vi "PWM-PID-ENCODER LIFA  - PID original  -Kalman filter test + PID  test new period of pid - Copie.vi"() -> ()   [LabVIEW 2018]
uses:
  <vilib>/LabVIEW Interface for Arduino/Type Defs/Board Type.ctl
  Control 1.ctl
  <vilib>/LabVIEW Interface for Arduino/Type Defs/Pin Mode.ctl
  <vilib>/Analysis/Matrix/Datatypes/RealMatrix.ctl
  <vilib>/addons/control/pid/pid.llb/PID (DBL).vi
  <vilib>/LabVIEW Interface for Arduino/LabVIEW Interface for Arduino.lvlib
  <vilib>/Analysis/Matrix/NI_Matrix.lvlib
  <vilib>/addons/control/pid/NI_PID_pid.lvlib
panel:
  in  "?":enum32{"Page 1", "Page 2"}(tab)
  in  "STOP":bool
  in  "RESET":bool
  in  "USB  COM":refnum<visa-resource-name>="COM12"
  in  "Platforme":T1
  in  "Direction 1":bool
  in  "Direction 2":bool
  in  "gains PID":T2={"Proportional gain (Kc)"=1.0, "Integral  (Ti )"=0.01, "Derivative  (Td)"=0.0} {"Derivative  (Td)" scale=0.0..30.0; "Integral  (Ti )" scale=0.0..30.0; "Proportional gain (Kc)" scale=0.0..30.0}
  in  "Consigne":dbl(knob) scale=0.0..1500.0
  out "PWM(%)":dbl(slide) scale=0.0..100.0
  out "Vitesse":T3
  in  "Contrôle manuel":dbl(knob) scale=100.0..255.0
  in  "Mode":bool
  out "Estimation de vitesse":cluster{"Real Matrix Element":dbl, dbl}(graph) caption="Waveform Chart"
  out "Vitesse  (tr/min)":dbl(knob) scale=0.0..1500.0
  # "Tableau de Bord"
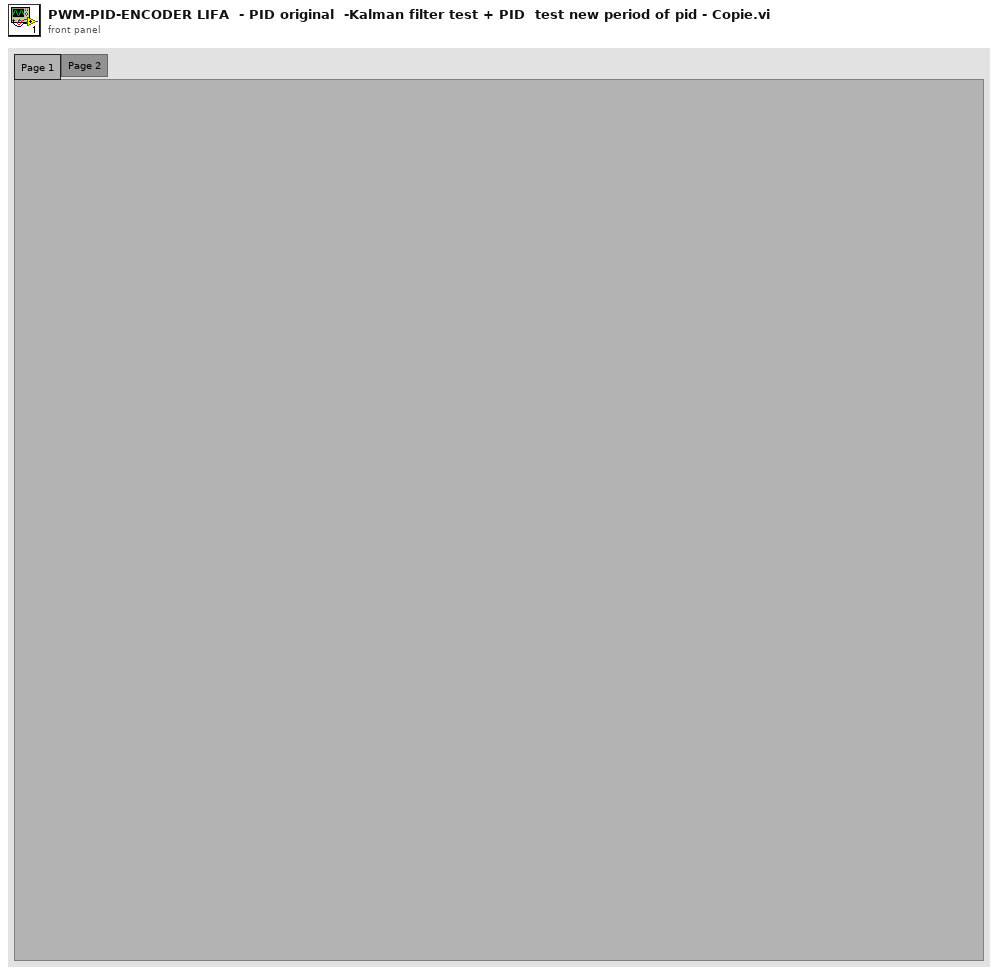
[diagram p1: front panel]
types:
  T1 = typedef "LabVIEW Interface for Arduino.lvlib/Board Type.ctl" = enum16{"Uno", "Dimuelanove w/Atmega 328", "Mega 2560"}
  T2 = cluster{"Proportional gain (Kc)":dbl, "Integral  (Ti )":dbl, "Derivative  (Td)":dbl}
  T3 = typedef "Control 1.ctl" = dynamicdata
  T4 = typedef "LabVIEW Interface for Arduino.lvlib/Pin Mode.ctl" = enum8{"Input", "Output"}
  T5 = typedef "LabVIEW Interface for Arduino.lvlib/Arduino Resource.ctl" = cluster{"VISA resource":refnum<visa-resource-name>, "Board Type":T1, "Connection Type":enum8{"USB / Serial"}, "Bytes Per Packet (15)":u8}
  T6 = typedef "NI_Matrix.lvlib/RealMatrix.ctl" = dbl[][]
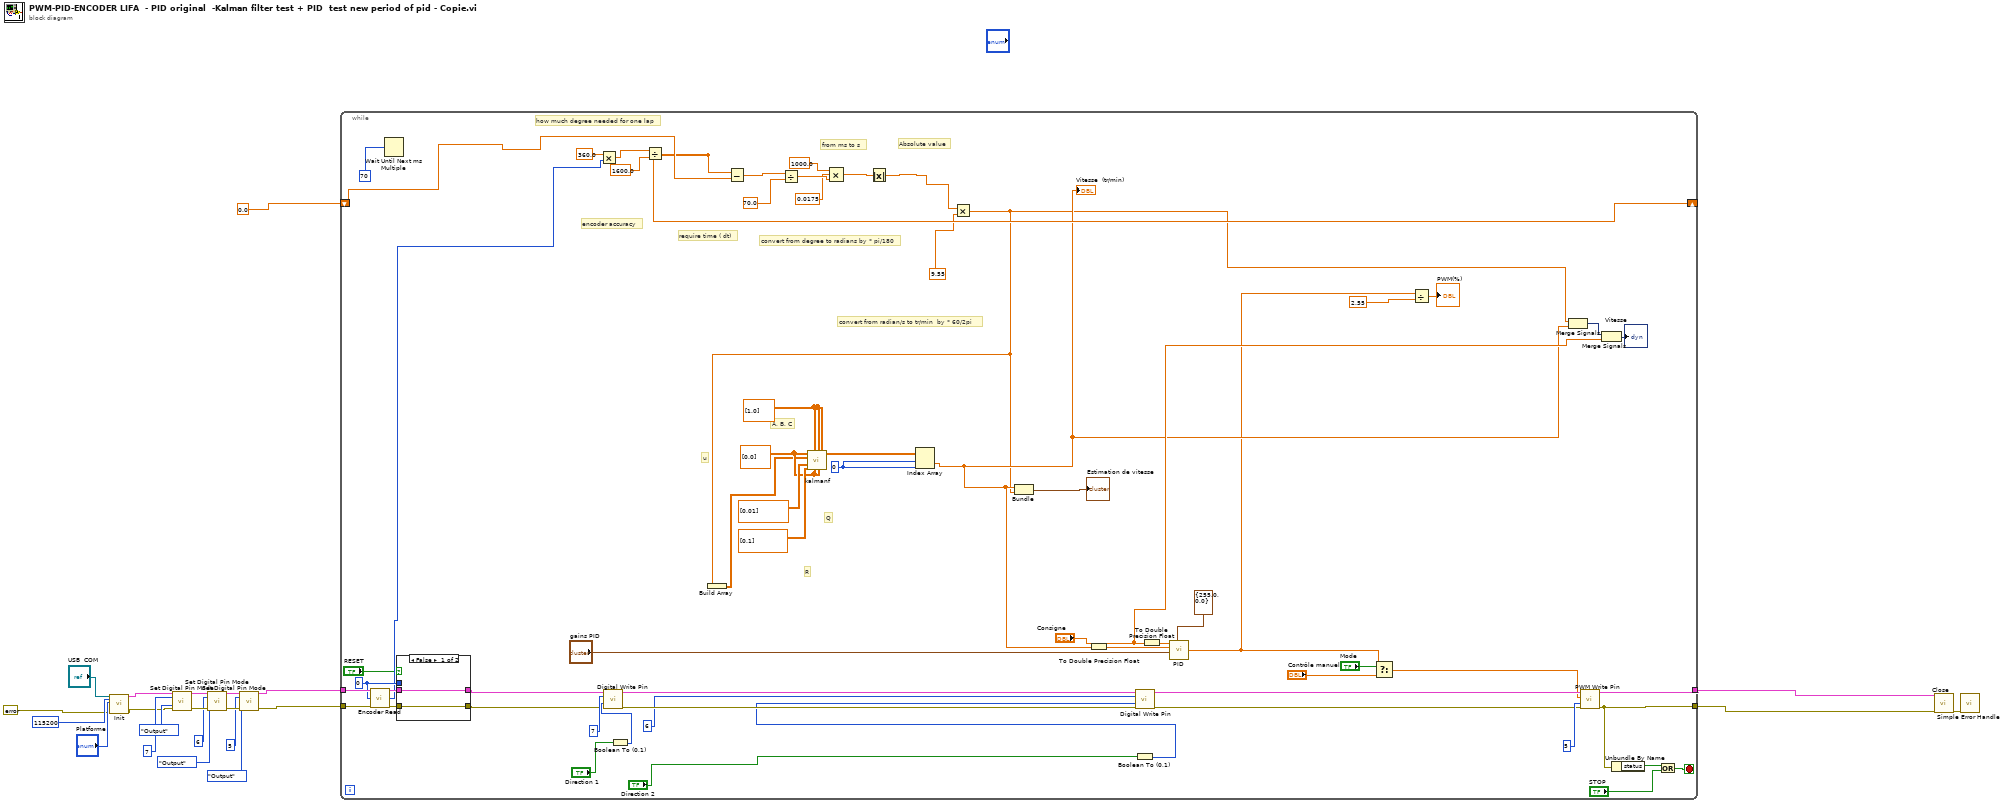
[diagram p0: block diagram]
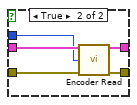
[diagram p2: hidden frame]
diagram:
  n1 = call <vilib>:"Init.vi"("VISA resource"="USB  COM", "Baud Rate (115200)"=u32 115200, "Board Type (Uno)"="Platforme", "error in"=errorcluster {"status"=FALSE, "code"=0, "source"=""}) -> ("Arduino Resource"=w7:T5, "error out"=w6:errorcluster)  [unwired: 14 in]
  n2 = call <vilib>:"Set Digital Pin Mode.vi"("Arduino Resource"=w7, "Digital I/O Pin"=u8 7, "Pin Mode (Input)"=Pin_Mode."Output", "error in"=w6) -> ("Arduino Resource"=w17:T5, "error out"=w16:errorcluster)  [unwired: 10 in]
  n3 = call <vilib>:"Set Digital Pin Mode.vi"("Arduino Resource"=w17, "Digital I/O Pin"=u8 6, "Pin Mode (Input)"=Pin_Mode."Output", "error in"=w16) -> ("Arduino Resource"=w15:T5, "error out"=w14:errorcluster)  [unwired: 10 in]
  n4 = call <vilib>:"Set Digital Pin Mode.vi"("Arduino Resource"=w15, "Digital I/O Pin"=u8 5, "Pin Mode (Input)"=Pin_Mode."Output", "error in"=w14) -> ("Arduino Resource"=w5:T5, "error out"=w4:errorcluster)  [unwired: 10 in]
  n5 = while {
    tunnel: w5 -> [w84]
    tunnel: w4 -> [w81]
    tunnel: [w64] -> w22
    tunnel: [w65] -> w2
    shift-right: [w29] -> _
    shift-left: 0.0 -> [w31]
    stop <- w80 stop-if-true
    w46 = 0 ("index (row)")
    w48 = T6 [[0.0]] ("U")
    w51 = T6 [[1.0]] ("A")
    w78 = u8 0 ("Encoder Number (0)")
    # "Absolute value"
    # "convert from radian/s to tr/min  by * 60/2pi"
    # "how much degree needed for one lap"
    # "encoder accuracy"
    # "from ms to s"
    # "require time ( dt)"
    # "convert from degree to radians by * pi/180"
    # "A, B, C"
    # "R"
    # "Q"
    # "u"
    n6 = call "Encoder Read.vi"("Arduino Resource"=w84, "Encoder Number (0)"=w78, "error in"=w81) -> ("Arduino Resource Out"=w83:T5, "Count"=w32:i32, "error out"=w82:errorcluster)  [unwired: 10 in]
    n7 = Wait Until Next ms Multiple(millisecond multiple=u32 70) -> ()  [unwired: 1 out]
    n8 = case shown="False" "RESET" {
      tunnel: w83 -> [w86 w91]
      tunnel: [w86 w90] -> w63
      tunnel: [w85 w89] -> w62
      tunnel: w82 -> [w85 w88]
      tunnel: w78 -> [_ w87]
      frame False {
      }
      frame True {
        n9 = call "Encoder Read.vi"("Arduino Resource"=w91, "Encoder Number (0)"=w87, "error in"=w88) -> ("Arduino Resource Out"=w90:T5, "error out"=w89:errorcluster)  [unwired: 10 in, 1 out]
      }
    }
    n10 = Multiply(x=360.0, y=w32) -> (x*y=w39:dbl)
    n11 = Boolean To (0,1)(Boolean="Direction 1") -> (0, 1=w69:i16)
    n12 = call <vilib>:"Digital Write Pin.vi"("Arduino Resource"=w63, "Digital I/O Pin (0)"=u8 7, "Value (0)"=w69, "error in"=w62) -> ("Arduino Resource"=w75:T5, "error out"=w74:errorcluster)  [unwired: 10 in]
    n13 = Divide(x=w39, y=1600.0) -> (x/y=w29:dbl)
    n14 = Subtract(x=w29, y=w31) -> (x-y=w37:dbl)
    n15 = Divide(x=w37, y=70.0) -> (x/y=w35:dbl)
    n16 = Compound Arithmetic op=MULTIPLY(1000.0 ("value"), 0.0175 ("value"), w35) -> (w28:dbl)
    n17 = Absolute Value(x=w28) -> (abs(x)=w26:dbl)
    n18 = Multiply(x=w26, y=9.55) -> (x*y=w24:dbl)
    n19 = Build Array(w24) -> (w47:T6)
    n20 = call "kalmanf.vi"("u"=w48, "A"=w51, "B"=w51, "C"=w51, "y"=w47, "Q"=T6 [[0.01]], "R"=T6 [[0.1]] ("Q"), "xhat0"=w48, "P0"=w48) -> ("xhat"=w45:T6)  [unwired: 6 in]
    n21 = Index Array(array=w45, index (row)=w46, index (col)=w46) -> (element=w25:dbl)
    "Vitesse  (tr/min)" <- w25
    n22 = Bundle("Real Matrix Element"=w25, w24) -> (→"Estimation de vitesse":cluster{"Real Matrix Element":dbl, dbl})  [unwired: 1 in]
    n23 = To Double Precision Float(number=w25) -> (double precision float=w59:dbl)
    n24 = Boolean To (0,1)(Boolean="Direction 2") -> (0, 1=w67:i16)
    n25 = call <vilib>:"Digital Write Pin.vi"("Arduino Resource"=w75, "Digital I/O Pin (0)"=u8 6, "Value (0)"=w67, "error in"=w74) -> ("Arduino Resource"=w73:T5, "error out"=w72:errorcluster)  [unwired: 10 in]
    n26 = To Double Precision Float(number="Consigne") -> (double precision float=w42:dbl)
    n27 = call-poly <vilib>:"PID.vi"("output range"=cluster{"output high":dbl, "output low":dbl} {"output high"=255.0, "output low"=0.0}, "PID gains"="gains PID", "process variable"=w59, "setpoint"=w42) -> ("output"=w23:dbl)  [unwired: 6 in, 1 out]
    n28 = Select(t=w23, s="Mode", f="Contrôle manuel") -> (s? t:f=w55:dbl)
    n29 = Divide(x=w23, y=2.55) -> (x/y=→"PWM(%)":dbl)
    n30 = Merge Signals(w24, w25) -> (w43:dynamicdata)
    n31 = call <vilib>:"PWM Write Pin.vi"("Arduino Resource"=w73, "Duty Cycle (0 - 255)"=w55, "PWM Pin (3)"=u8 5, "error in"=w72) -> ("Arduino Resource"=w64:T5, "error out"=w65:errorcluster)  [unwired: 10 in]
    n32 = Merge Signals(w43, "Consigne") -> (→"Vitesse":dynamicdata)
    n33 = Unbundle By Name(w65) -> ("status"=w79:bool)
    n34 = Or(x=w79, y="STOP") -> (x .or. y?=w80:bool)
  }
  n35 = call <vilib>:"Close.vi"("Arduino Resource"=w22, "error in"=w2) -> ("error out"=w21:errorcluster)  [unwired: 13 in]
  n36 = call <vilib>:"Simple Error Handler.vi"("error in (no error)"=w21) -> ()  [unwired: 4 in, 5 out]
